vi "TxPkt - Handle Port Channel.vi"(8 "error in (no error)":errorcluster, 11 "Packet Ref in":T1 format="%.0x") -> (0 "error out":errorcluster, 3 "Packet Ref out":T1 format="%.0x")   [LabVIEW 2019, in "UDP-Custom-Device System Explorer.lvlib"]
uses:
  UDP-Custom-Device System Explorer.lvlib
  <vilib>/NI VeriStand/Custom Device API/Custom Device Item Ref.ctl
  <vilib>/NI VeriStand/Custom Device API/Custom Device Channel.ctl
  <vilib>/NI VeriStand/Custom Device API/Custom Device Channel Type.ctl
  <vilib>/NI VeriStand/Custom Device Tools/Custom Device Utility Library/NI VeriStand - Search for Item by Name.vi
  <vilib>/NI VeriStand/Custom Device API/Custom Device API.lvlib
  Property Accessors/Tx Packet Accessors.lvlib
  <vilib>/NI VeriStand/Custom Device Tools/Custom Device Utility Library/Custom Device Utility Library.lvlib
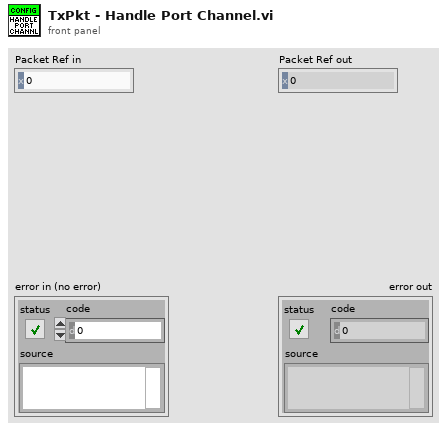
[diagram p1: front panel]
types:
  T1 = typedef "Custom Device API.lvlib/Custom Device Item Ref.ctl" = u64
  T2 = typedef "Custom Device API.lvlib/Custom Device Channel.ctl" = cluster{"Type":T3, "Units":string, "Default Value":dbl, "Faultable":bool, "Scalable":bool}
  T3 = typedef "Custom Device API.lvlib/Custom Device Channel Type.ctl" = enum16{"Input", "Output"}
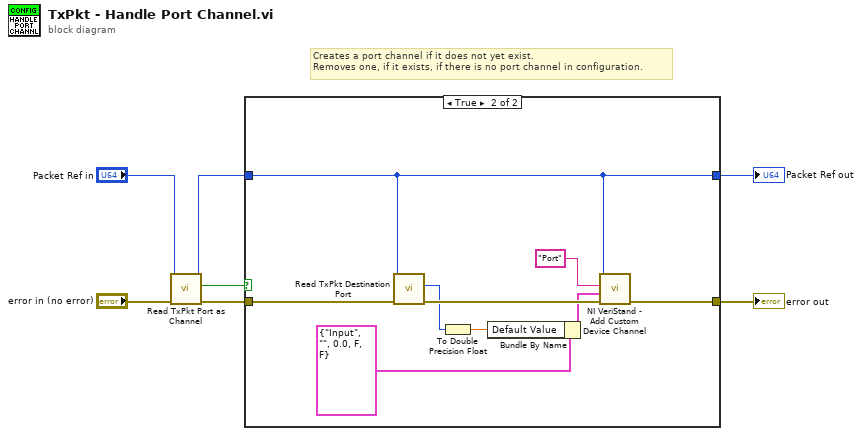
[diagram p0: block diagram]
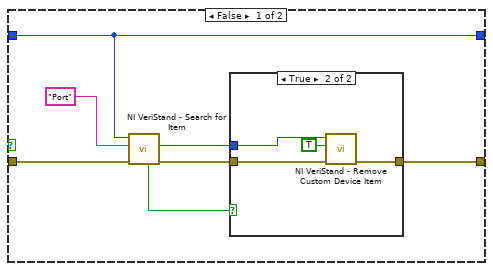
[diagram p2: hidden frame]
diagram:
  # "Creates a port channel if it does not yet exist.\nRemoves one, if it exists, if there is no port channel in configuration."
  n1 = call "Read TxPkt Port as Channel.vi"("error in (no error)"="error in (no error)", "Node Ptr"="Packet Ref in") -> ("error out"=w2:errorcluster, "Port as Channel"=w1:bool, "Node Ptr out"=w4:T1)  [unwired: 7 in]
  n2 = case shown="True" w1 {
    tunnel: w2 -> [w13 w25]
    tunnel: w4 -> [w8 w26]
    tunnel: [w11 w28] -> w7
    tunnel: [w8 w26] -> w6
    frame False {
      n3 = call-poly <vilib>:"NI VeriStand - Search for Item.vi"("error in"=w13, "Item Name"="Port", "Section Ref in"=w8) -> ("error out"=w12:errorcluster, "Item Ref"=w9:T1, "Found"=w10:bool)  [unwired: 5 in, 1 out]
      n4 = case shown="True" w10 {
        tunnel: w12 -> [w15 w19]
        tunnel: [w15 w18] -> w11
        tunnel: w9 -> [_ w17]
        frame False {
        }
        frame True {
          n5 = call <vilib>:"NI VeriStand - Remove Custom Device Item.vi"("error in (no error)"=w19, "Force Delete (F)"=TRUE, "Item Ref in"=w17) -> ("error out"=w18:errorcluster)  [unwired: 7 in, 1 out]
        }
      }
    }
    frame True {
      n6 = call "Read TxPkt Destination Port.vi"("error in (no error)"=w25, "Node Ptr"=w26) -> ("error out"=w24:errorcluster, "Destination Port"=w21:u16)  [unwired: 7 in, 1 out]
      n7 = To Double Precision Float(number=w21) -> (double precision float=w20:dbl)
      n8 = Bundle By Name(cluster=T2 {"Type"=enum."Input", "Units"="", "Default Value"=0.0, "Faultable"=FALSE, "Scalable"=FALSE} ("Channel"), "Default Value"=w20) -> (w22:T2)
      n9 = call <vilib>:"NI VeriStand - Add Custom Device Channel.vi"("error in (no error)"=w24, "Channel"=w22, "Channel Name"="Port", "Parent Ref in"=w26) -> ("error out"=w28:errorcluster)  [unwired: 4 in, 3 out]
    }
  }
  "error out" <- w7
  "Packet Ref out" <- w6
